vi "GetNumberOfColumns.vi"(4 "error in (no error)":errorcluster, 7 "Matching Nodes":refnum<k20>[](array[refnum])) -> (0 "error out":errorcluster, 3 "#Columns":i32)   [LabVIEW 2013, in "Spreadsheet.lvclass"]
uses:
  Spreadsheet.lvclass
  XML.lvlib
  <resource>/objmgr/DOMUserDefRef.rc
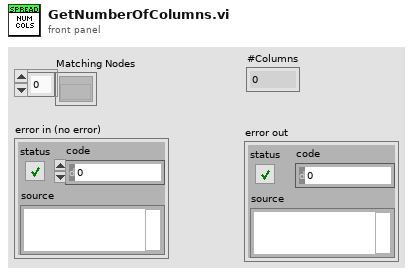
[diagram p1: front panel]
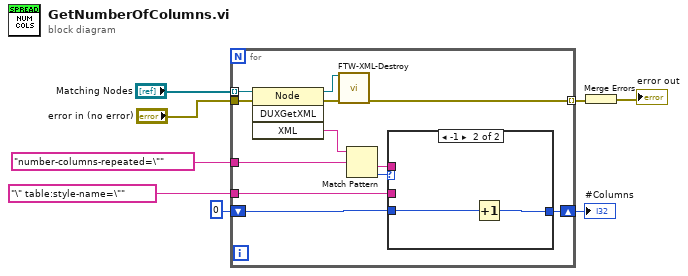
[diagram p0: block diagram]
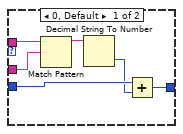
[diagram p2: hidden frame]
diagram:
  n1 = for {
    tunnel: "Matching Nodes" -> [w20] mode=indexing
    tunnel: "error in (no error)" -> [w19]
    tunnel: "number-columns-repeated=\"" -> [w15]
    shift-right: [w14] -> w1
    shift-left: 0 -> [w13]
    tunnel: "\" table:style-name=\"" -> [w10]
    tunnel: [w9] -> w2 mode=indexing
    n2 = invoke class="Node" method="DUXGetXML"(reference=w20, error in=w19) -> (reference out=w17:refnum<k20>, error out=w18:errorcluster, "XML"=w16:string)  [unwired: 2 in, 1 out]
    n3 = call "FTW-XML-Destroy.vi"("XML Node"=w17, "error in"=w18) -> ("error out"=w9:errorcluster)  [unwired: 13 in]
    n4 = Match Pattern(string=w16, regular expression=w15) -> (after substring=w12:string, offset past match=w11:i32)  [unwired: 1 in, 2 out]
    n5 = case shown="-1" w11 {
      tunnel: w13 -> [w22 w28]
      tunnel: [w23 w27] -> w14
      tunnel: w12 -> [w26 _]
      tunnel: w10 -> [w25 _]
      frame 0, Default {
        n6 = Match Pattern(string=w26, regular expression=w25) -> (before substring=w24:string)  [unwired: 1 in, 3 out]
        n7 = Decimal String To Number(string=w24) -> (number=w21:i32)  [unwired: 2 in, 1 out]
        n8 = Add(x=w22, y=w21) -> (x+y=w23:i32)
      }
      frame -1 {
        n9 = Increment(x=w28) -> (x+1=w27:i32)
      }
    }
  }
  "#Columns" <- w1
  n10 = Merge Errors(w2) -> (→"error out":errorcluster)
